vi "validate configuration.vi"(8 "error in":errorcluster, 11 "configuration in":refnum<class "PL_Target Configuration.lvclass">) -> (0 "error out":errorcluster, 3 "configuration out":refnum<class "PL_Target Configuration.lvclass">)   [LabVIEW 2013, in "PL_Target Configuration.lvclass"]
doc: "Provides an interface for performing validation on a given configuration. Any children should define the behavior of this function to ensure that the configuration in memory can be used by the runtime class."
uses:
  PL_Target Configuration.lvclass
  <vilib>/NI/Tag Bus Module Framework/root configuration/TBM configuration.lvclass
  PL_Target Configuration.lvclass/PL_Target Configuration.ctl
  <vilib>/NI/CEF/CEF_TreeControl/NISE_CEF_TreeControl.lvlib
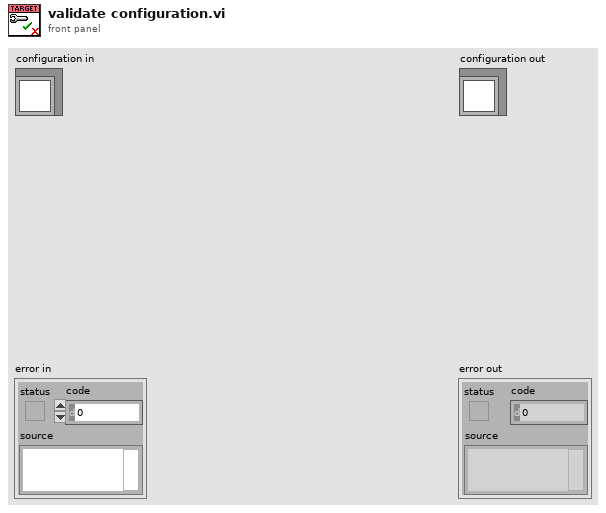
[diagram p1: front panel]
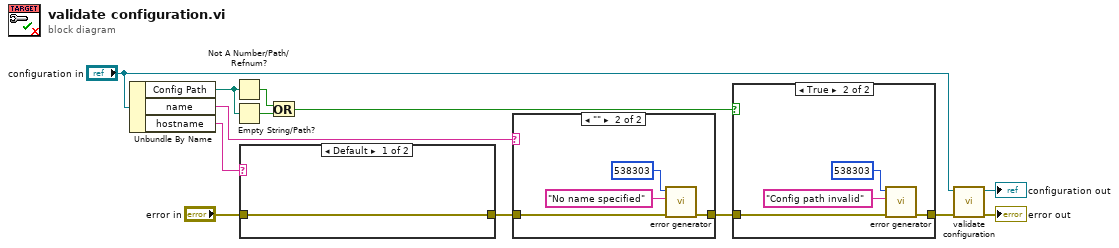
[diagram p0: block diagram]
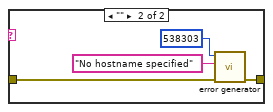
[diagram p2: hidden frame]
diagram:
  n1 = Unbundle By Name("configuration in") -> ("Config Path"=w4:path, "name"=w10:string, "hostname"=w1:string)
  n2 = Not A Number/Path/Refnum?(number/path/refnum=w4) -> (NaN/Path/Refnum?=w8:bool)
  n3 = Empty String/Path?(string/path=w4) -> (empty?=w9:bool)
  n4 = case shown="Default" w1 {
    tunnel: [w14 w17] -> w3
    tunnel: "error in" -> [w14 w18]
    frame Default {
    }
    frame "" {
      n5 = call <vilib>:"error generator.vi"("error in"=w18, "append error message"="No hostname specified" ("error message (\"\")"), "error code (0)"=538303) -> ("error out"=w17:errorcluster)  [unwired: 6 in]
    }
  }
  n6 = Or(x=w8, y=w9) -> (x .or. y?=w7:bool)
  n7 = case shown="\"\"" w10 {
    tunnel: [w19 w23] -> w5
    tunnel: w3 -> [w19 w20]
    frame Default {
    }
    frame "" {
      n8 = call <vilib>:"error generator.vi"("error in"=w20, "append error message"="No name specified" ("error message (\"\")"), "error code (0)"=538303) -> ("error out"=w23:errorcluster)  [unwired: 6 in]
    }
  }
  n9 = case shown="True" w7 {
    tunnel: [w24 w26] -> w6
    tunnel: w5 -> [w24 w27]
    frame False {
    }
    frame True {
      n10 = call <vilib>:"error generator.vi"("error in"=w27, "append error message"="Config path invalid" ("error message (\"\")"), "error code (0)"=538303) -> ("error out"=w26:errorcluster)  [unwired: 6 in]
    }
  }
  n11 = call-parent "validate configuration.vi"("error in"=w6, "configuration in"="configuration in") -> ("error out"=→"error out":errorcluster, "configuration out"=→"configuration out":refnum<class "PL_Target Configuration.lvclass">)  [unwired: 8 in]
